vi "Write Hardware Configuration.vi"(8 "error in":errorcluster, 10 "path":path, 11 "custom device":T1 format="%.0x") -> (0 "error out":errorcluster, 3 "custom device out":T1 format="%.0x")   [LabVIEW 2020, in "Ballard ARINC 429 Hardware Configuration.lvlib"]
uses:
  Ballard ARINC 429 Hardware Configuration.lvlib
  <vilib>/NI VeriStand/Custom Device API/Custom Device Item Ref.ctl
  <vilib>/NI VeriStand/Custom Device API/Custom Device API.lvlib
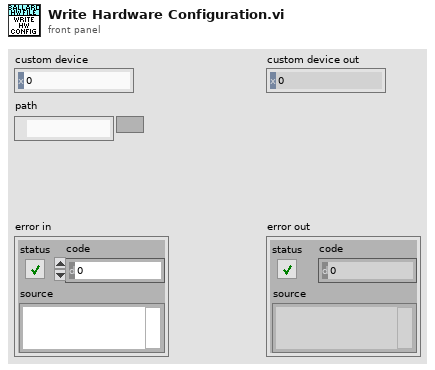
[diagram p1: front panel]
types:
  T1 = typedef "Custom Device API.lvlib/Custom Device Item Ref.ctl" = u64
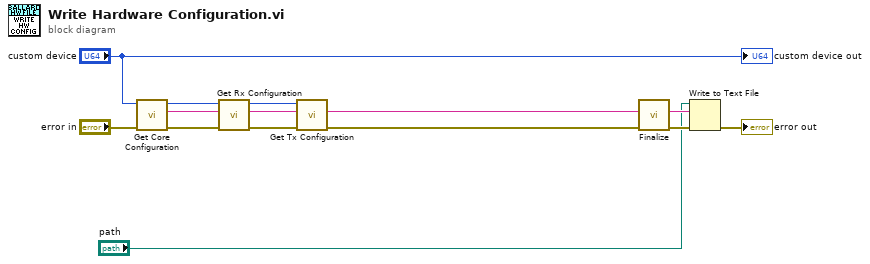
[diagram p0: block diagram]
diagram:
  n1 = call "Get Core Configuration.vi"("error in"="error in", "custom device"="custom device") -> ("error out"=w8:errorcluster, "configuration string"=w6:string, "custom device out"=w7:T1)  [unwired: 7 in]
  n2 = call "Get Rx Configuration.vi"("error in"=w8, "configuration string"=w6, "custom device"=w7) -> ("error out"=w5:errorcluster, "configuration string out"=w2:string, "custom device out"=w1:T1)  [unwired: 6 in]
  n3 = call "Get Tx Configuration.vi"("error in"=w5, "configuration string"=w2, "custom device"=w1) -> ("error out"=w4:errorcluster, "configuration string out"=w3:string)  [unwired: 6 in, 1 out]
  n4 = call "Finalize.vi"("error in"=w4, "configuration string"=w3) -> ("error out"=w12:errorcluster, "configuration string out"=w11:string)  [unwired: 8 in]
  n5 = Write to Text File(file (use dialog)="path", text=w11, error in=w12) -> (error out=→"error out":errorcluster)  [unwired: 1 in, 2 out]
  "custom device out" <- "custom device"
